vi "Interpolation (Control - Window Init Mem - Graph) Test.vi"() -> ()   [LabVIEW 2014]
uses:
  <vilib>/FPGAPlugInAG/sbRIO-9636/niLvFpga_Open_sbRIO-9636.vi
  <vilib>/rvi/interface/common/dynamic/niFpgaDynamicAddResources.vi
  <vilib>/Utility/error.llb/Error Cluster From Error Code.vi
  <vilib>/rvi/errors/niLvFpgaAdjustHostInterfaceError.vi
  <vilib>/rvi/interface/common/niFpgaWaitOnOcc.vi
  <vilib>/FPGAPlugInAG/Dynamic/niLvFpga_Run_Dynamic.vi
  <vilib>/FPGAPlugInAG/Dynamic/niLvFpga_Abort_Dynamic.vi
  <vilib>/FPGAPlugInAG/Dynamic/niLvFpga_Close_Dynamic.vi
  <vilib>/rvi/interface/nirviOpenFPGA/nirviOpenFPGA.xnode
  FPGA Bitfiles/LaserDistanceSen_FPGATarget_DoubleFFTMesuram_3A9FBl7sWYY.lvbitx
  FPGA Target/Test VIs/Double FFT Mesurament (Max Bin detection - Control - Windowing - Graph) test.vi
  <vilib>/rvi/interface/nirviReadWriteControl/nirviReadWriteControl.xnode
  <vilib>/rvi/interface/nirviMethod/nirviMethod.xnode
  <vilib>/rvi/interface/nirviCloseFPGA/nirviCloseFPGA.xnode
  <vilib>/FPGAPlugInAG/Dynamic/niLvFpga_ConfigureFifo_Dynamic.vi
  <vilib>/rvi/errors/niLvFpgaMergeErrorWithErrorCode.vi
  <vilib>/FPGAPlugInAG/Dynamic/niLvFpga_StartFifo_Dynamic.vi
  <vilib>/rvi/interface/Simulation/niFpgaSimulationCallBeginRW.vi
  NiFpgaLv.dll
  <vilib>/FPGAPlugInAG/Dynamic/niLvFpga_ReadFifo_Dynamic.vi
panel:
  out "FFT (freq)":waveform(dbl)(graph)
  out "Signal (points)":dbl[](graph)
  out "Signal (t)":waveform(dbl)(graph)
  out "FFT (bin)":dbl[](graph)
  in  "Snapshot":bool
  out "Ftone+":dbl
  out "Ftone-":dbl
  in  "Windowing":T1(ring)
  in  "first bin":i32=10
  in  "last bin":i32=255
  in  "lower limit 2":u32(slide)=677 scale=625.0..737.0
  in  "lower limit 1":u32(slide)=59 scale=0.0..112.0
  out "Detected Frequency Tone - (Hz)":dbl
  in  "stop":bool
  out "Max Bin":i32
  out "Max Amp":dbl format="%.2f"
  out "Prev Bin":i32
  out "Next Bin":i32
  out "Prev Amp":dbl format="%.2f"
  out "Next Amp":dbl format="%.2f"
  out "Interpolated Bin":dbl
  in  "Interpolation Method":T2(ring)
  # "WARNING:\nOnce pressed wait untill the end of operation"
  # "ONLINE parameter"
  # "OFFLINE parameters"
  # "Max Detection FFT bin range"
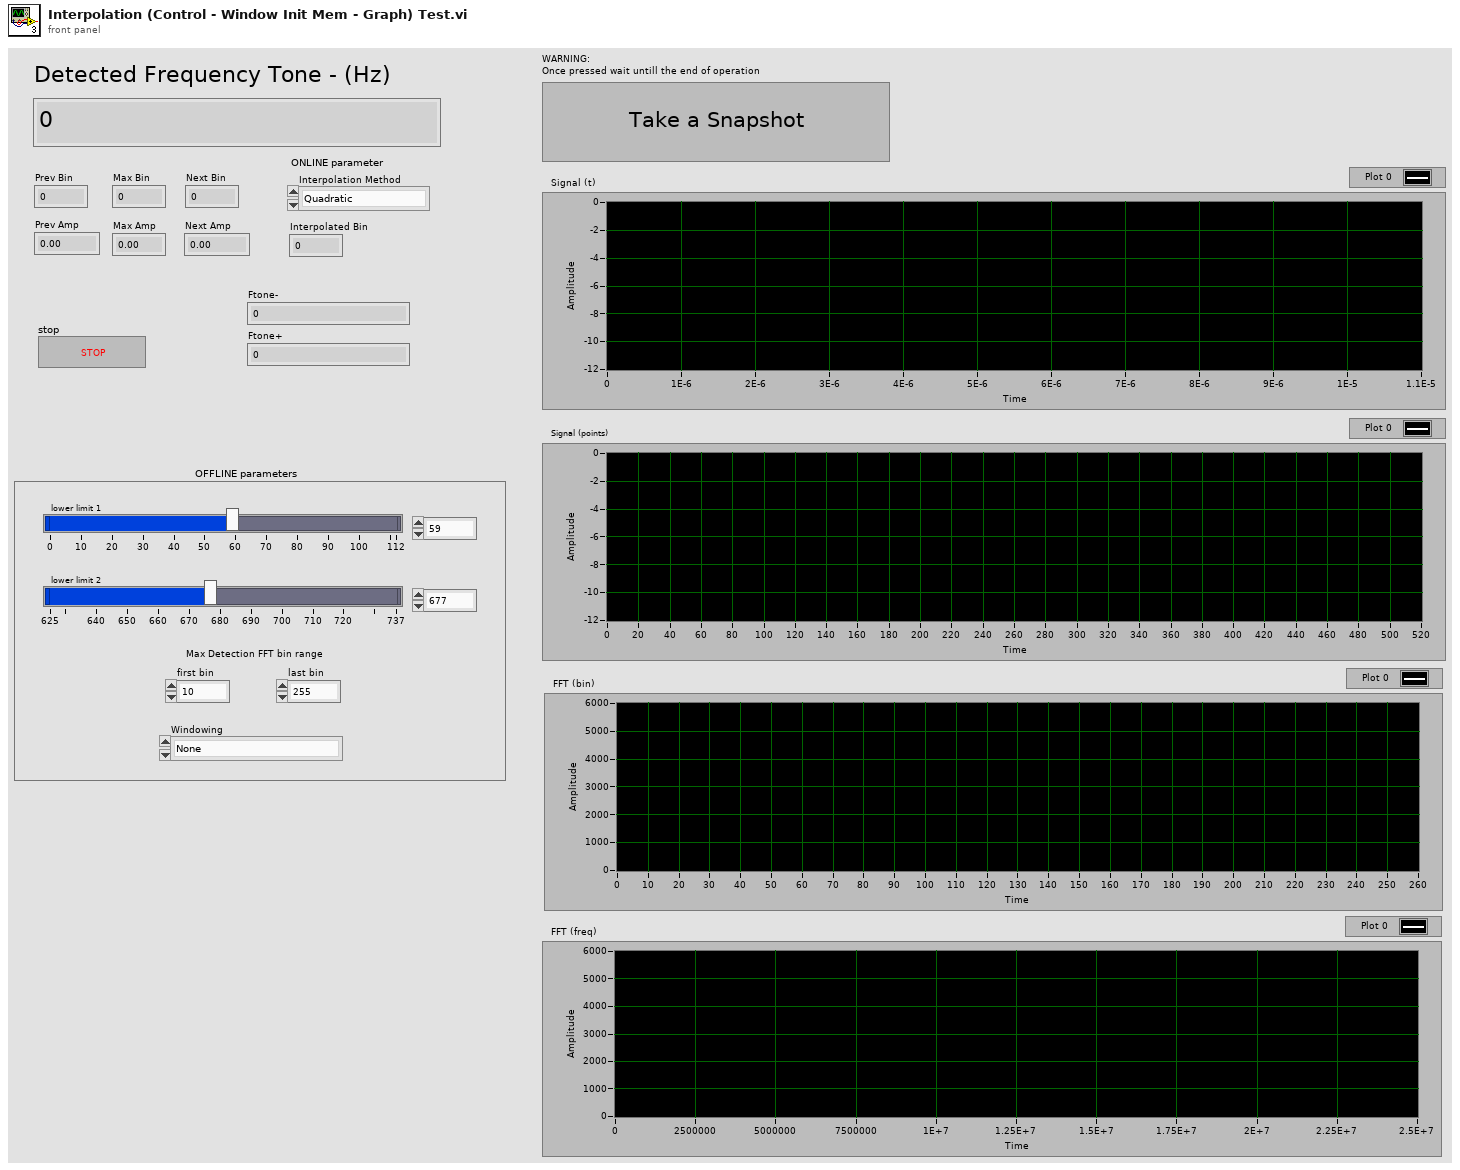
[diagram p1: front panel]
types:
  T1 = enum16{"None", "Hanning", "Hamming", "Blackman", "Blackman-Harris"}
  T2 = enum16{"Quadratic", "McLeodd", "Barycentric", "Jain"}
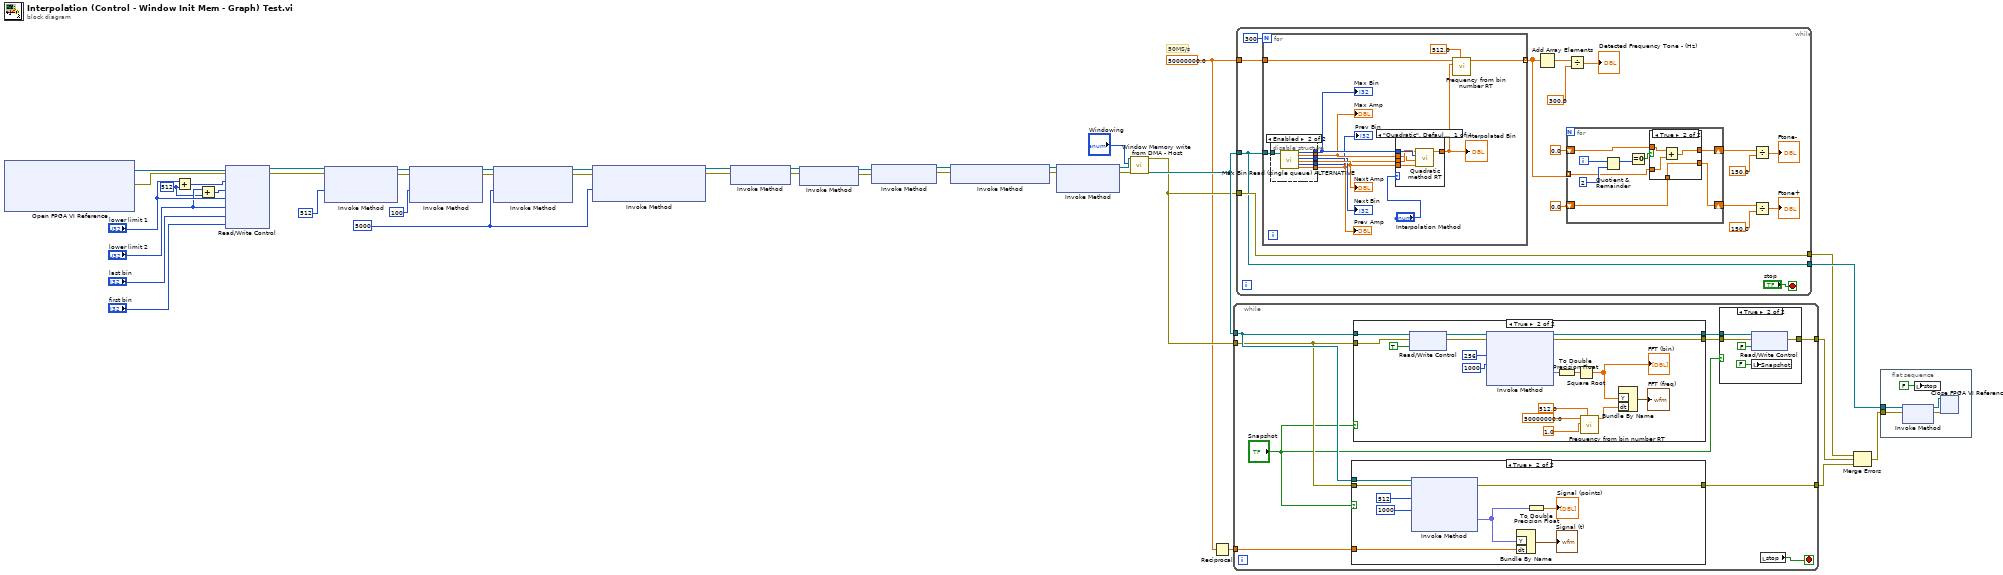
[diagram p0: block diagram]
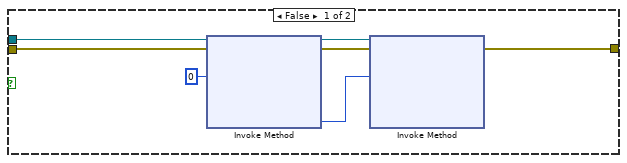
[diagram p3: hidden frame]
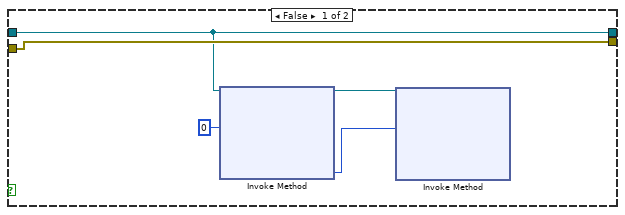
[diagram p4: hidden frame]
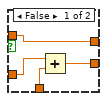
[diagram p5: hidden frame]
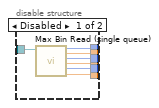
[diagram p6: hidden frame]
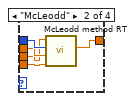
[diagram p7: hidden frame]
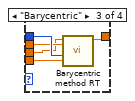
[diagram p8: hidden frame]
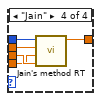
[diagram p9: hidden frame]
diagram:
  w34 = u32 512 ("y")
  w1 = 50000000.0 ("Sample Rate (S/s)")
  w18 = u32 5000 ("Requested Depth")
  # "50MS/s"
  n1 = xnode "Open FPGA VI Reference"() -> ("FPGA VI Reference Out"=w33:refnum<k20>, "error out"=w32:errorcluster)  [unwired: 2 in]
  n2 = Add(x="lower limit 1", y=w34) -> (x+y=w38:u32)
  n3 = Add(x="lower limit 2", y=w34) -> (x+y=w36:u32)
  n4 = xnode "Read/Write Control"("FPGA VI Reference In"=w33, "error in"=w32, "upper limit 1"=w38, "upper limit 2"=w36, "lower limit 1"="lower limit 1", "lower limit 2"="lower limit 2", "last bin"="last bin", "first bin"="first bin") -> ("FPGA VI Reference Out"=w26:refnum<k20>, "error out"=w25:errorcluster)
  n5 = xnode "Invoke Method"("FPGA VI Reference In"=w26, "error in"=w25, "Requested Depth"=u32 512) -> ("FPGA VI Reference Out"=w24:refnum<k20>, "error out"=w23:errorcluster)  [unwired: 1 out]
  n6 = xnode "Invoke Method"("FPGA VI Reference In"=w24, "error in"=w23, "Requested Depth"=u32 100) -> ("FPGA VI Reference Out"=w22:refnum<k20>, "error out"=w21:errorcluster)  [unwired: 1 out]
  n7 = xnode "Invoke Method"("FPGA VI Reference In"=w22, "error in"=w21, "Requested Depth"=w18) -> ("FPGA VI Reference Out"=w20:refnum<k20>, "error out"=w19:errorcluster)  [unwired: 1 out]
  n8 = xnode "Invoke Method"("FPGA VI Reference In"=w20, "error in"=w19, "Requested Depth"=w18) -> ("FPGA VI Reference Out"=w11:refnum<k20>, "error out"=w10:errorcluster)  [unwired: 1 out]
  n9 = xnode "Invoke Method"("FPGA VI Reference In"=w11, "error in"=w10) -> ("FPGA VI Reference Out"=w13:refnum<k20>, "error out"=w12:errorcluster)
  n10 = xnode "Invoke Method"("FPGA VI Reference In"=w13, "error in"=w12) -> ("FPGA VI Reference Out"=w15:refnum<k20>, "error out"=w14:errorcluster)
  n11 = xnode "Invoke Method"("FPGA VI Reference In"=w15, "error in"=w14) -> ("FPGA VI Reference Out"=w9:refnum<k20>, "error out"=w8:errorcluster)
  n12 = xnode "Invoke Method"("FPGA VI Reference In"=w9, "error in"=w8) -> ("FPGA VI Reference Out"=w7:refnum<k20>, "error out"=w27:errorcluster)
  n13 = xnode "Invoke Method"("FPGA VI Reference In"=w7, "error in"=w27) -> ("FPGA VI Reference Out"=w41:refnum<k20>, "error out"=w42:errorcluster)  [unwired: 1 in]
  n14 = call "Window Memory write from DMA - Host.vi"("error in"=w42, "Enum"="Windowing", "FPGA VI Reference In"=w41) -> ("FPGA VI Reference Out"=w29:refnum<k20>, "error out"=w28:errorcluster)  [unwired: 5 in, 2 out]
  n15 = Reciprocal(x=w1) -> (1/x=w2:dbl)
  n16 = while {
    tunnel: w29 -> [w51]
    tunnel: w28 -> [w50]
    tunnel: [w47] -> w6
    tunnel: [w46] -> w5
    tunnel: w2 -> [w44]
    stop <- w49 stop-if-true
    n17 = case shown="True" "Snapshot" {
      tunnel: w51 -> [w63 w73]
      tunnel: w50 -> [w61 w72]
      tunnel: [w60 w69] -> w46
      tunnel: w44 -> [_ w67]
      frame False {
        n18 = xnode "Invoke Method"("FPGA VI Reference In"=w63, "error in"=w61, "Number of Elements"=u32 0) -> ("FPGA VI Reference Out"=w59:refnum<k20>, "error out"=w58:errorcluster, "Elements Remaining"=w62:u32)  [unwired: 1 in, 1 out]
        n19 = xnode "Invoke Method"("FPGA VI Reference In"=w59, "error in"=w58, "Number of Elements"=w62) -> ("error out"=w60:errorcluster)  [unwired: 1 in, 3 out]
      }
      frame True {
        n20 = xnode "Invoke Method"("FPGA VI Reference In"=w73, "error in"=w72, "Number of Elements"=u32 512, "Timeout (ms)"=1000) -> ("error out"=w69:errorcluster, "Data"=w66:fxp<+/-,12,12>[])  [unwired: 2 out]
        n21 = Bundle By Name("Y"=w66, "dt"=w67) -> (→"Signal (t)":waveform(dbl))  [unwired: 1 in]
        n22 = To Double Precision Float(number=w66) -> (double precision float=→"Signal (points)":dbl[])
      }
    }
    n23 = case shown="True" "Snapshot" {
      tunnel: w51 -> [w76 w95]
      tunnel: w50 -> [w78 w94]
      tunnel: [w78 w93] -> w48
      tunnel: [w76 w92] -> w45
      frame False {
        n24 = xnode "Invoke Method"("FPGA VI Reference In"=w76, "Number of Elements"=u32 0) -> ("FPGA VI Reference Out"=w74:refnum<k20>, "Elements Remaining"=w75:u32)  [unwired: 2 in, 2 out]
        n25 = xnode "Invoke Method"("FPGA VI Reference In"=w74, "Number of Elements"=w75) -> ()  [unwired: 2 in, 4 out]
      }
      frame True {
        n26 = xnode "Read/Write Control"("FPGA VI Reference In"=w95, "error in"=w94, "snapshot"=TRUE) -> ("FPGA VI Reference Out"=w90:refnum<k20>, "error out"=w89:errorcluster)
        n27 = xnode "Invoke Method"("FPGA VI Reference In"=w90, "error in"=w89, "Number of Elements"=u32 256, "Timeout (ms)"=1000) -> ("FPGA VI Reference Out"=w92:refnum<k20>, "error out"=w93:errorcluster, "Data"=w86:fxp<+,44,44>[])  [unwired: 1 out]
        n28 = To Double Precision Float(number=w86) -> (double precision float=w85:dbl[])
        n29 = Square Root(x=w85) -> (sqrt(x)=w80:dbl[])
        "FFT (bin)" <- w80
        n30 = call "Frequency from bin number RT.vi"("FFT size"=512.0, "Bin number"=1.0, "Sample Rate (S/s)"=50000000.0) -> ("Detected Frequency (Hz)"=w81:dbl)  [unwired: 8 in]
        n31 = Bundle By Name("Y"=w80, "dt"=w81) -> (→"FFT (freq)":waveform(dbl))  [unwired: 1 in]
      }
    }
    n32 = case shown="True" "Snapshot" {
      tunnel: w48 -> [w52 w57]
      tunnel: [w52 w56] -> w47
      tunnel: w45 -> [_ w55]
      frame False {
      }
      frame True {
        n33 = xnode "Read/Write Control"("FPGA VI Reference In"=w55, "error in"=w57, "snapshot"=FALSE) -> ("error out"=w56:errorcluster)  [unwired: 1 out]
        n34 = local write "Snapshot"(FALSE ("Snapshot")) -> ()
      }
    }
    n35 = local read "stop"() -> (w49:bool)
  }
  n36 = while {
    tunnel: w1 -> [w111]
    tunnel: w29 -> [w96]
    tunnel: w28 -> [w97]
    tunnel: [w96] -> w31
    tunnel: [w97] -> w4
    stop <- "stop" stop-if-true
    n37 = for {
      N: 300 -> [_]
      tunnel: w96 -> [w136]
      tunnel: w111 -> [w139]
      tunnel: [w137] -> w103 mode=indexing
      n38 = disable-structure shown="Enabled" {
        disable-tunnel: w136 -> [w148 w155]
        disable-tunnel: [w147 w154] -> w135
        disable-tunnel: [w146 w153] -> w134
        disable-tunnel: [w145 w151] -> w133
        disable-tunnel: [w144 w149] -> w132
        disable-tunnel: [w143 w150] -> w131
        disable-tunnel: [w142 w152] -> w130
        frame Disabled {
          n39 = call "Max Bin Read (single queue).vi"("FPGA VI Reference In"=w148) -> ("Max Bin"=w147:i32, "Max Amp"=w146:dbl, "Next Bin"=w142:i32, "Next Amp"=w145:dbl, "Prev Bin"=w143:i32, "Prev Amp"=w144:dbl)  [unwired: 13 in]
        }
        frame Enabled {
          n40 = call "Max Bin Read (single queue) ALTERNATIVE.vi"("FPGA VI Reference In"=w155) -> ("Max Bin"=w154:i32, "Max Amp"=w153:dbl, "Next Bin"=w152:i32, "Next Amp"=w151:dbl, "Prev Bin"=w150:i32, "Prev Amp"=w149:dbl)  [unwired: 13 in]
        }
      }
      "Max Bin" <- w135
      "Max Amp" <- w134
      "Prev Bin" <- w131
      "Next Bin" <- w130
      "Prev Amp" <- w132
      "Next Amp" <- w133
      n41 = case shown="\"Quadratic\", Default" "Interpolation Method" {
        tunnel: w135 -> [w159 w164 w169 w174]
        tunnel: w134 -> [w156 w163 w168 w173]
        tunnel: w132 -> [w157 w162 w167 w172]
        tunnel: w133 -> [w158 w161 w166 w171]
        tunnel: [w160 w165 w170 w175] -> w138
        frame "Quadratic", Default {
          n42 = call "Quadratic method RT.vi"("Next Amplitude"=w158, "Max Amplitude"=w156, "Max bin"=w159, "Prev Amplitude"=w157) -> ("Bin"=w160:dbl)  [unwired: 7 in]
        }
        frame "McLeodd" {
          n43 = call "McLeodd method RT.vi"("Next Amp"=w161, "Max Amp"=w163, "Max Bin"=w164, "Prev Amp"=w162) -> ("Bin"=w165:dbl)  [unwired: 7 in]
        }
        frame "Barycentric" {
          n44 = call "Barycentric method RT.vi"("Next Amp"=w166, "Max Bin"=w169, "Max Amp"=w168, "Prev Amp"=w167) -> ("Bin"=w170:dbl)  [unwired: 7 in]
        }
        frame "Jain" {
          n45 = call "Jain's method RT.vi"("Prev Amp"=w172, "Next Amp"=w171, "Max Amp"=w173, "Max Bin"=w174) -> ("Bin"=w175:dbl)  [unwired: 7 in]
        }
      }
      "Interpolated Bin" <- w138
      n46 = call "Frequency from bin number RT.vi"("FFT size"=512.0, "Bin number"=w138, "Sample Rate (S/s)"=w139) -> ("Detected Frequency (Hz)"=w137:dbl)  [unwired: 8 in]
    }
    n47 = Add Array Elements(numeric array=w103) -> (sum=w110:dbl)
    n48 = for {
      tunnel: w103 -> [w116] mode=indexing
      shift-right: [w115] -> w106
      shift-left: 0.0 -> [w117]
      shift-right: [w113] -> w99
      shift-left: 0.0 -> [w114]
      i -> [w121]
      n49 = Quotient & Remainder(x=w121, y=2) -> (x-y*floor(x/y)=w119:i32)  [unwired: 1 out]
      n50 = Equal To 0?(x=w119) -> (x = 0?=w118:bool)
      n51 = case shown="True" w118 {
        tunnel: w117 -> [w125 w129]
        tunnel: w116 -> [w124 w128]
        tunnel: [w125 w127] -> w115
        tunnel: w114 -> [w123 w126]
        tunnel: [w122 w126] -> w113
        frame False {
          n52 = Add(x=w124, y=w123) -> (x+y=w122:dbl)
        }
        frame True {
          n53 = Add(x=w129, y=w128) -> (x+y=w127:dbl)
        }
      }
    }
    n54 = Divide(x=w110, y=300.0) -> (x/y=→"Detected Frequency Tone - (Hz)":dbl)
    n55 = Divide(x=w106, y=150.0) -> (x/y=→"Ftone-":dbl)
    n56 = Divide(x=w99, y=150.0) -> (x/y=→"Ftone+":dbl)
  }
  n57 = Merge Errors(w4, w6, w5) -> (w3:errorcluster)
  n58 = flat-sequence {
    tunnel: w31 -> [w178]
    tunnel: w3 -> [w177]
    frame #0 {
      n59 = xnode "Invoke Method"("FPGA VI Reference In"=w178, "error in"=w177) -> ("FPGA VI Reference Out"=w179:refnum<k20>, "error out"=w180:errorcluster)
      n60 = local write "stop"(FALSE ("stop")) -> ()
      n61 = xnode "Close FPGA VI Reference"("FPGA VI Reference In"=w179, "error in"=w180) -> ()  [unwired: 1 out]
    }
  }
